vi "DFConfig Search Area.vi"(8 "error in (no error)":errorcluster, 9 "Datafinder Search Area":T1={"path"=path "C:/Program Files/Summitek/Spartan/data/TDM", "remotepath"=path "C:/Program Files/Summitek/Spartan/data/TDM", "alias"="Spartan", "volatile"=TRUE, "type"="favorite", "lastcrawl"=timestamp(0 s since 1904-01-01), "numberofcrawls"=0, "crawlnow"=TRUE}, 10 "CrawlDir ID (\"\")":string, 11 "My.DataFinder In":string) -> (0 "error out":errorcluster, 3 "My.DataFinder Out":string)   [LabVIEW 2011]
uses:
  DFConfig SEARCH AREA.ctl
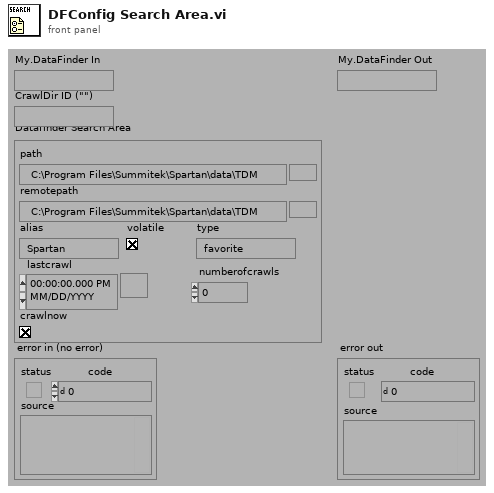
[diagram p1: front panel]
types:
  T1 = typedef "DFConfig SEARCH AREA.ctl" = cluster{"path":path, "remotepath":path, "alias":string, "volatile":bool, "type":string, "lastcrawl":timestamp, "numberofcrawls":i32, "crawlnow":bool}
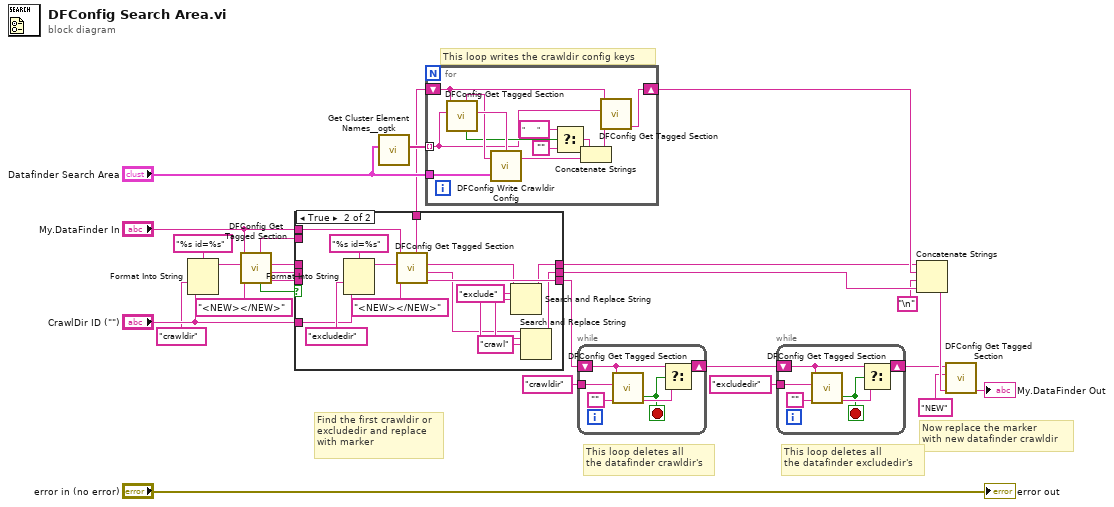
[diagram p0: block diagram]
diagram:
  # "This loop deletes all\nthe datafinder excludedir's"
  # "Now replace the marker\nwith new datafinder crawldir"
  # "Find the first crawldir or\nexcludedir and replace\nwith marker"
  # "This loop deletes all\nthe datafinder crawldir's"
  # "This loop writes the crawldir config keys"
  n1 = Format Into String(format string="%s id=%s", "crawldir" ("Tag (\"\")"), "CrawlDir ID (\"\")") -> (resulting string=w26:string)  [unwired: 2 in, 1 out]
  n2 = call "DFConfig Get Tagged Section.vi"("Replacement String (\"\")"="<NEW></NEW>", "Tag (\"\")"=w26, "String"="My.DataFinder In") -> ("String with Replacement"=w16:string, "End Tag"=w15:string, "Start Tag"=w14:string, "Not Found?"=w17:bool, "InnerString"=w9:string)  [unwired: 4 out]
  n3 = case shown="True" w17 {
    tunnel: w16 -> [w29 _]
    tunnel: w15 -> [w30 _]
    tunnel: w14 -> [w31 _]
    tunnel: [w31 w33] -> w13
    tunnel: [w30 w32] -> w12
    tunnel: [w29 w40] -> w11
    tunnel: "My.DataFinder In" -> [_ w42]
    tunnel: w9 -> [w28 _]
    tunnel: [w28 w41] -> w8
    tunnel: "CrawlDir ID (\"\")" -> [_ w38]
    frame False {
    }
    frame True {
      w37 = "crawl" ("replace string (\"\")")
      w36 = "exclude" ("search string")
      n4 = Format Into String(format string="%s id=%s", "excludedir" ("Tag (\"\")"), w38) -> (resulting string=w43:string)  [unwired: 2 in, 1 out]
      n5 = call "DFConfig Get Tagged Section.vi"("Replacement String (\"\")"="<NEW></NEW>", "Tag (\"\")"=w43, "String"=w42) -> ("String with Replacement"=w40:string, "End Tag"=w35:string, "Start Tag"=w34:string, "InnerString"=w41:string)  [unwired: 5 out]
      n6 = Search and Replace String(input string=w34, search string=w36, replace string=w37) -> (result string=w33:string)  [unwired: 1 in, 7 out]
      n7 = Search and Replace String(input string=w35, search string=w36, replace string=w37) -> (result string=w32:string)  [unwired: 1 in, 7 out]
    }
  }
  n8 = call "Get Cluster Element Names__ogtk.vi"("Cluster"="Datafinder Search Area") -> ("Element Names"=w20:string[])  [unwired: 1 in, 9 out]
  n9 = for {
    tunnel: w20 -> [w49] mode=indexing
    shift-right: [w53] -> w19
    shift-left: w8 -> [w54]
    tunnel: "Datafinder Search Area" -> [w56]
    n10 = call "DFConfig Get Tagged Section.vi"("Tag (\"\")"=w49, "String"=w54) -> ("Start Tag"=w57:string, "Not Found?"=w50:bool, "InnerString"=w55:string)  [unwired: 1 in, 6 out]
    n11 = call "DFConfig Write Crawldir Config.vi"("Datafinder Search Area"=w56, "Config In"=w55, "Tag (\"\")"=w57) -> ("Config Out"=w52:string)  [unwired: 2 out]
    n12 = Select(t="      ", s=w50, f="") -> (s? t:f=w46:string)
    n13 = Concatenate Strings(w46, w52) -> (w51:string)
    n14 = call "DFConfig Get Tagged Section.vi"("Replacement String (\"\")"=w51, "Tag (\"\")"=w49, "String"=w54) -> ("String with Replacement"=w53:string)  [unwired: 8 out]
  }
  n15 = while {
    shift-right: [w62] -> w4
    shift-left: w11 -> [w61]
    tunnel: "crawldir" ("Tag (\"\")") -> [w58]
    stop <- w59 stop-if-true
    n16 = call "DFConfig Get Tagged Section.vi"("Replacement String (\"\")"="", "Tag (\"\")"=w58, "String"=w61) -> ("String with Replacement"=w60:string, "Not Found?"=w59:bool)  [unwired: 7 out]
    n17 = Select(t=w61, s=w59, f=w60) -> (s? t:f=w62:string)
  }
  n18 = while {
    shift-right: [w68] -> w3
    shift-left: w4 -> [w67]
    tunnel: "excludedir" ("Tag (\"\")") -> [w64]
    stop <- w65 stop-if-true
    n19 = call "DFConfig Get Tagged Section.vi"("Replacement String (\"\")"="", "Tag (\"\")"=w64, "String"=w67) -> ("String with Replacement"=w66:string, "Not Found?"=w65:bool)  [unwired: 7 out]
    n20 = Select(t=w67, s=w65, f=w66) -> (s? t:f=w68:string)
  }
  n21 = Concatenate Strings(w13, w19, "\n", w12) -> (w24:string)
  n22 = call "DFConfig Get Tagged Section.vi"("Replacement String (\"\")"=w24, "Tag (\"\")"="NEW", "String"=w3) -> ("String with Replacement"=→"My.DataFinder Out":string)  [unwired: 8 out]
  "error out" <- "error in (no error)"
